vi "Tutorial 02.vi"() -> ()   [LabVIEW 2014]
panel:
  out "Result":dbl
  in  "Numeric 4":dbl=3.0
  in  "Numeric 3":dbl=8.0
  in  "Numeric 2":dbl=10.0
  in  "Numeric":dbl=5.0
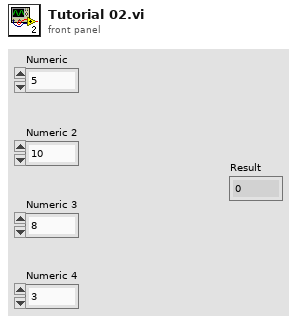
[diagram p1: front panel]
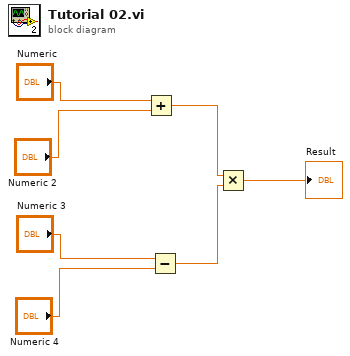
[diagram p0: block diagram]
diagram:
  n1 = Add(x="Numeric", y="Numeric 2") -> (x+y=w2:dbl)
  n2 = Subtract(x="Numeric 3", y="Numeric 4") -> (x-y=w3:dbl)
  n3 = Multiply(x=w2, y=w3) -> (x*y=→"Result":dbl)
